vi "Neslab Comm Demo.vi"() -> ()   [LabVIEW 2016]
doc: "For new users, one must run MAX, and have it search for Devices and Interfaces. Once it finds the comm port you are using for the chiller(s), it will be available in the VISA Resource Name control on the front panel, where you must choose it before running the vi. This VI is a demo, showing how to use the Neslab Comm vi, and is not intended to be used as a subvi within a larger program. \n\nIt first opens a VISA serial port, which could be either RS-232, 422, or 485, and tests the comm port with a request for acknowledge. It then starts a while loop, continuously polling for the chiller internal temperature, and on demand, setting or reading any of the chiller parameters. In the Comm vi, the choice of Set/Read action command is made using an enumerated type input. We wrote this and tested it only with RS232 comms with two chillers, each on it's own USB COM port converter. If simultaneous calls are being made, the comm subvi needs to be made re-entrant using the checkbox in VI properties. \n\nSome of the binary encoding/decoding from the previously posted driver was recycled, decimal parsing corrected, and the checksum calculation simplified using the method mentioned in the Neslab manual. \n\nReporting of checksum errors through the Error Cluster output is optional, controlled by Report Cksum Error boolean control. When this is set to OFF, device dependent comm errors with the chiller will be ignored, and the inpossible value 666 will be reported as output value. This allows the main DAQ application to continue running when the chiller is turned off. This assumes that the VISA comm port is still working. Visa errors indicating a problem with the serial port will still be reported.\n\nCare should be taken not to inadvertently change the PID tuning parameters, which can render the unit inoperable. If this should happen, the factory default parameters are listed in the chiller manual, and there is a procedure to return all defaults from the setup menu via the chiller front panel.\n\nAlso, take care not to adjust the setpoint below the freezing point of the coolant. Don't wreck your chiller!\n\nBill Gilbert, 1-01-2019"
panel:
  out "Instructions":string="For new users, one must run MAX, and have it search for Devices and Interfaces. Once it finds the comm port you are using for the chiller(s), it will be available in the VISA Resource Name control on the front panel, where you must choose it before running the vi. This VI is a demo, showing how to use the Neslab Comm vi, and is not intended to be used as a subvi within a larger program.  \n\nIt first opens a VISA serial port, which could be either RS-232, 422, or 485, and tests the comm port with a request for acknowledge. It  then starts a while loop, continuously polling for the chiller internal temperature, and on demand, setting or reading any of the chiller parameters. \n\nSome of the code from the previously posted driver was recycled, corrected, and the cheksum calculation was  simplified using the method mentioned in the Neslab manual. \n\nCare should be taken not to inadvertently change the PID tuning parameters, which can render the unit inoperable. If this should happen, the factory default parameters are listed in the chiller manual, and there is a procedure to return all defaults from the setup menu via the chiller front panel.\n\nAlso, take care not to adjust the setpoint below the freezing point of the coolant.\n\nBill Gilbert, 1-01-2019"
  in  "Poll mS":u32=500
  in  "Send Command":bool
  out "read buffer 2":string
  out "read buffer 1":string
  out "Internal Temp":dbl format="%.2f"
  in  "Report Cksm Err":bool=TRUE
  in  "Serial Settings":T1={"baud rate"=9600, "data bits"=8, "stop bits"=10, "parity"=enum."None", "flow control"=0, "TermChar Enable"=TRUE, "Term Char "=10} {"Term Char" format="%02x"; "flow control" items=["None", "XON/XOFF", "RTS/CTS", "XON/XOFF & RTS/CTS", "DTR/DSR", "XON/XOFF & DTR/DSR"]; "stop bits" items=["1.0"=10, "1.5"=15, "2.0"=20]; "data bits" min=5 max=8 step=1}
  out "error out":errorcluster
  out "Description":string
  out "Value":dbl format="%.2f"
  in  "Readback mS":u32=100
  in  "Value to Set":dbl=20.0
  in  "Command":T2(ring)
  in  "Exit":bool
  in  "timeout mS":u32=1000
  in  "VISA resource name":refnum<visa-resource-name>="COM4"
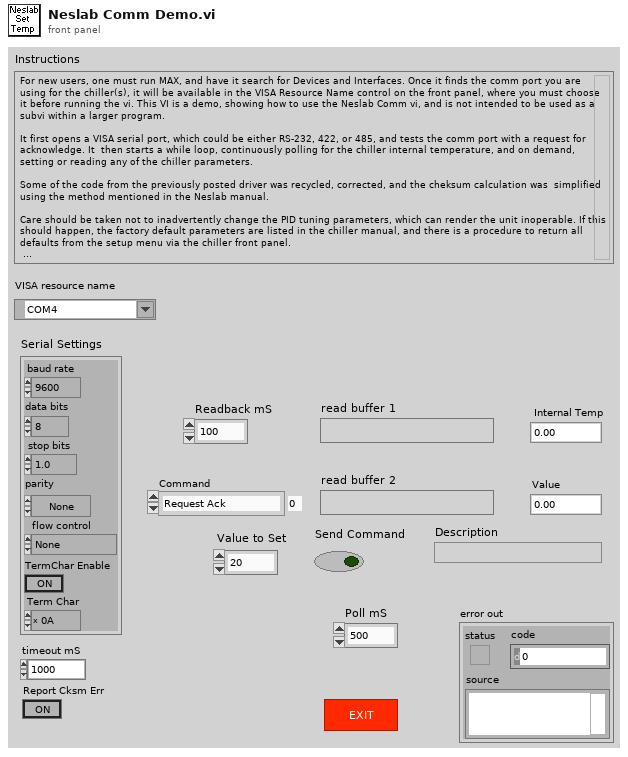
[diagram p1: front panel]
types:
  T1 = cluster{"baud rate":u32, "data bits":u16, "stop bits":u16, "parity":enum16{"None", "Odd", "Even", "Mark", "Space"}, "flow control":u16, "TermChar Enable":bool, "Term Char ":u8}
  T2 = enum16{"Request Ack", "Set Setpoint", "Set Lo Limit", "Set Hi Limit", "Set Prop Band 0-99.9", "Set Integral 0-9.99", "Set Derivative 0-5.0", "Read Int Temp", "Read Ext Temp", "Read Setpoint", "Read Low Limit", "Read High Limit", "Read Prop Band", "Read Integral", "Read Derivative "}
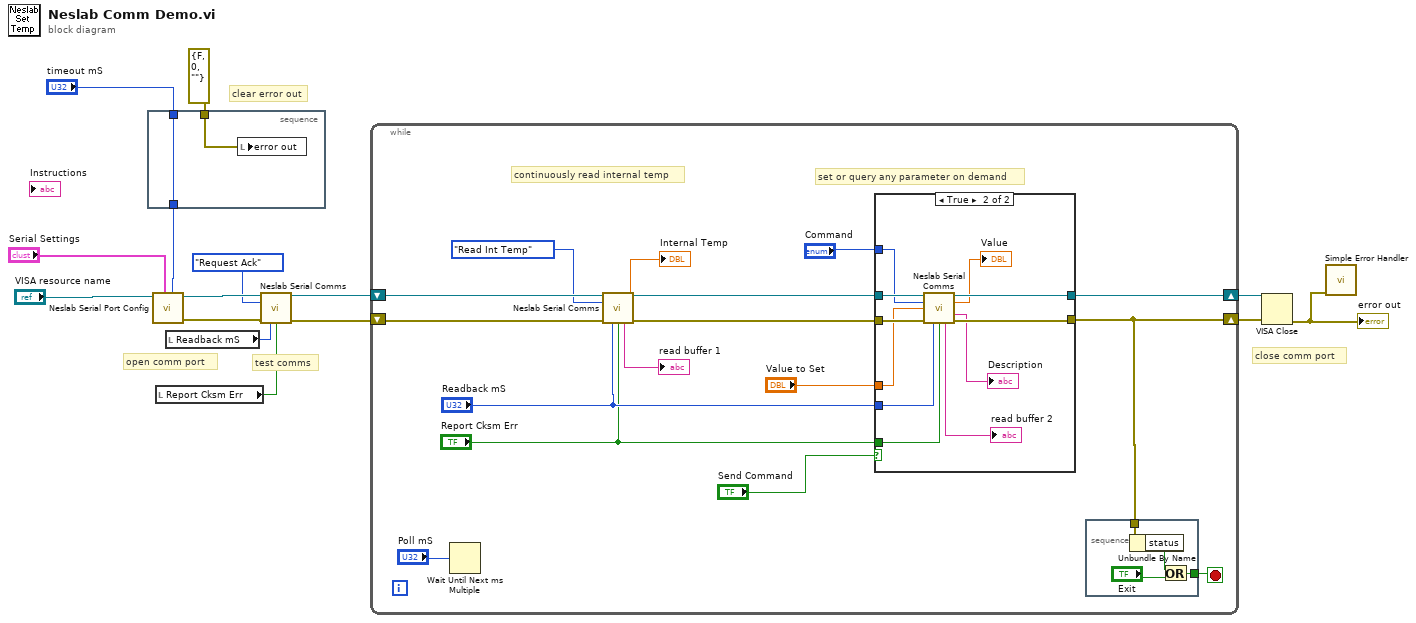
[diagram p0: block diagram]
diagram:
  # "clear error out"
  # "close comm port"
  # "test comms"
  # "open comm port"
  n1 = stacked-sequence {
    tunnel: [w17] -> w9
    tunnel: "timeout mS" -> [w17]
    tunnel: errorcluster {"status"=FALSE, "code"=0, "source"=""} ("error out") -> [w16]
    frame #0 {
      n2 = local write "error out"(w16) -> ()
    }
  }
  n3 = call <userlib>:"Neslab Serial Port Config.vi"("timeout mS"=w9, "Serial Settings"="Serial Settings", "VISA resource name"="VISA resource name") -> ("error out"=w6:errorcluster, "VISA out"=w7:refnum<visa-resource-name>)  [unwired: 5 in]
  n4 = local read "Report Cksm Err"() -> (w1:bool)
  n5 = local read "Readback mS"() -> (w2:u32)
  n6 = call <userlib>:"Neslab Serial Comms.vi"("VISA resource name"=w7, "Command"=T2."Request Ack", "error in"=w6, "Readback wait mS"=w2, "Report Cksm Err"=w1) -> ("VISA out"=w3:refnum<visa-resource-name>, "error out"=w4:errorcluster)  [unwired: 4 in, 5 out]
  n7 = while {
    shift-right: [w32] -> w14
    shift-left: w4 -> [w27]
    shift-right: [w33] -> w13
    shift-left: w3 -> [w28]
    stop <- w31 stop-if-true
    # "set or query any parameter on demand"
    # "continuously read internal temp"
    n8 = Wait Until Next ms Multiple(millisecond multiple="Poll mS") -> ()  [unwired: 1 out]
    n9 = call <userlib>:"Neslab Serial Comms.vi"("VISA resource name"=w28, "Command"=T2."Read Int Temp" ("Command 2"), "error in"=w27, "Readback wait mS"="Readback mS", "Report Cksm Err"="Report Cksm Err") -> ("VISA out"=w26:refnum<visa-resource-name>, "Numeric\nValue"=→"Internal Temp":dbl, "read buffer (hex)"=→"read buffer 1":string, "error out"=w25:errorcluster)  [unwired: 4 in, 3 out]
    n10 = case shown="True" "Send Command" {
      tunnel: w25 -> [w39 w49]
      tunnel: [w39 w46] -> w32
      tunnel: w26 -> [w38 w50]
      tunnel: [w38 w45] -> w33
      tunnel: "Value to Set" -> [_ w48]
      tunnel: "Command" -> [_ w47]
      tunnel: "Readback mS" -> [_ w42]
      tunnel: "Report Cksm Err" -> [_ w40]
      frame False {
      }
      frame True {
        n11 = call <userlib>:"Neslab Serial Comms.vi"("VISA resource name"=w50, "Command"=w47, "Set Value"=w48, "error in"=w49, "Readback wait mS"=w42, "Report Cksm Err"=w40) -> ("VISA out"=w45:refnum<visa-resource-name>, "Numeric\nValue"=→"Value":dbl, "Description"=→"Description":string, "read buffer (hex)"=→"read buffer 2":string, "error out"=w46:errorcluster)  [unwired: 3 in, 2 out]
      }
    }
    n12 = stacked-sequence {
      tunnel: w32 -> [w37]
      tunnel: [w34] -> w31
      frame #0 {
        n13 = Unbundle By Name(w37) -> ("status"=w36:bool)
        n14 = Or(x=w36, y="Exit") -> (x .or. y?=w34:bool)
      }
    }
  }
  n15 = VISA Close(VISA resource name=w13, error in (no error)=w14) -> (error out=w12:errorcluster)
  "error out" <- w12
  n16 = call <vilib>:"Simple Error Handler.vi"("error in (no error)"=w12) -> ()  [unwired: 1 in, 8 out]
